vi "ICS Structure.vi"() -> ()   [LabVIEW 2018]
panel:
  in  "EXIT":bool
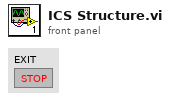
[diagram p1: front panel]
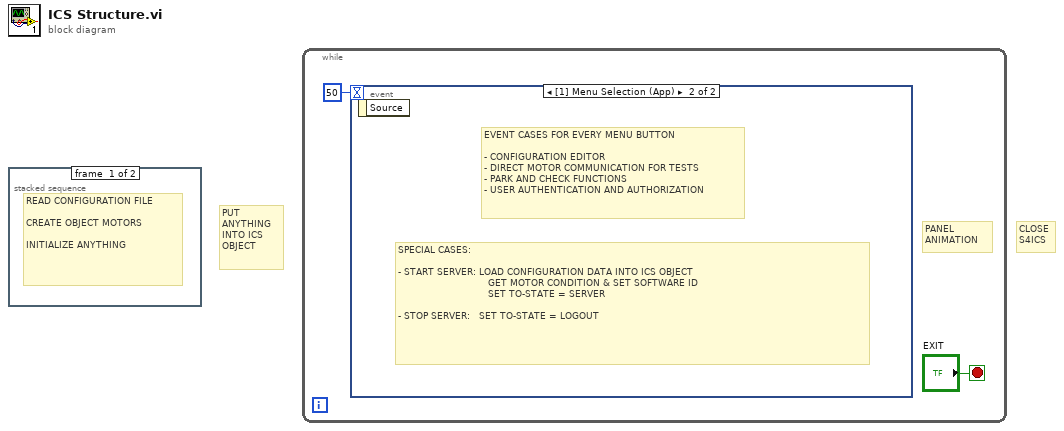
[diagram p0: block diagram]
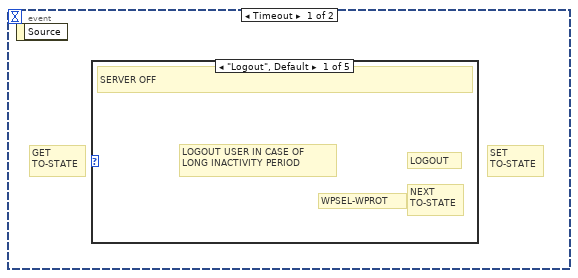
[diagram p2: hidden frame]
diagram:
  # "CLOSE\nS4ICS"
  # "PUT ANYTHING\nINTO ICS OBJECT"
  n1 = stacked-sequence {
    frame #0 {
      # "READ CONFIGURATION FILE\n\nCREATE OBJECT MOTORS\n\nINITIALIZE ANYTHING"
    }
    frame #1 {
    }
  }
  n2 = while {
    stop <- "EXIT" stop-if-true
    # "PANEL\nANIMATION"
    n3 = event shown="[1] Menu Selection (App)" {
      selector: _ -> [_ _]
      dyn-events: _ -> [_ _]
      timeout: 50 -> [_ _]
      event Timeout {
        # "SET\nTO-STATE"
        # "GET\nTO-STATE"
        n4 = event-data() -> ()  [unwired: 1 in, 1 out]
        n5 = case shown="\"Logout\", Default" {
          selector: _ -> [_ _ _ _ _]
          frame "Logout", Default {
            # "WPSEL-WPROT"
            # "NEXT\nTO-STATE"
            # "LOGOUT"
            # "LOGOUT USER IN CASE OF \nLONG INACTIVITY PERIOD"
            # "SERVER OFF"
          }
          frame "Server" {
            # "NEXT\nTO-STATE"
            # "LISTEN, READ CMD,\nSEND STATUS."
            # "CHECK FOR COMMAND"
          }
          frame "WPSEL-WPOT" {
            # "NEXT\nTO-STATE"
            # "CALW-ASEL"
            # "SERVER"
            # "IF MOVING, UPDATE STATUS\nIF CMD RECEIVED, SEND INSTRUCTIONS"
          }
          frame "GMIR-GFOC" {
            # "WPSEL-WPROT"
            # "NEXT\nTO-STATE"
            # "IF MOVING, UPDATE STATUS\nIF CMD RECEIVED, SEND INSTRUCTIONS"
            # "SERVER"
          }
          frame "CALW-ASEL" {
            # "GMIR-GFOC"
            # "NEXT\nTO-STATE"
            # "IF MOVING, UPDATE STATUS\nIF CMD RECEIVED, SEND INSTRUCTIONS"
            # "SERVER"
          }
        }
      }
      event Menu Selection (App) {
        # "SPECIAL CASES:\n\n- START SERVER: LOAD CONFIGURATION DATA INTO ICS OBJECT\n                              GET MOTOR CONDITION & SET SOFTWARE ID\n                              SET TO-STATE = SERVER\n\n- STOP SERVER:   SET TO-STATE = LOGOUT"
        # "EVENT CASES FOR EVERY MENU BUTTON\n\n- CONFIGURATION EDITOR\n- DIRECT MOTOR COMMUNICATION FOR TESTS\n- PARK AND CHECK FUNCTIONS\n- USER AUTHENTICATION AND AUTHORIZATION"
        n6 = event-data() -> ()  [unwired: 1 in, 1 out]
      }
    }
  }
